vi "NetworkUDP_Recieve.vi"(8 "error in (no error)":errorcluster, 9 "timeout ms (25000)":i32=25000, 10 "IP4 address":u32, 11 "receiver port":u16=5801) -> (0 "error out":errorcluster, 1 "UDP Network Connection out":refnum<k16>, 2 "ConsecErrCount":i32, 3 "data out":string, 4 "SenderAddress":u32)   [LabVIEW 2019, in "Trajectory_Library.lvlib"]
doc: "Listen for and read a packet of data from the network using the UDP protocol. This routine can listen for a single computer or listen for any senders on the subnet. \n\nThis subVI does not return to the caller until either data has been received or a timeout has occured. Suggest putting this function in a separate loop to avoid issues slowing down other code.\n\nInputs:\n -- Receiver Port -- UInt16 -- UDP port number used for listening. Only data sent to this port will be returned. (Optional. Default: 5801)\n -- IP4 Address -- UInt32 -- The IP address of the computer expected to send data. If this value is 0, then then data will be returned for any sender. Use the standard TCP/IP LabVIEW functions to convert a standard IP4 address in the form of 123.123.123.123 to an unsigned integer for this input. (Optional. Default: 0) \n -- Timeout ms -- Int32 -- Timeout value in milliseconds. (Optional. Default: 25000 )\n -- Error in -- Error cluster -- Propagated error cluster. (Optional. Default: no error)\n\nOutputs:\n -- data out -- string -- Last data message sent to the specified port number.\n -- Consec Err -- Int32 -- Counter indicating the number of consecutive errors that have occured.\n -- UDP Network Connection -- UDP Connection Reference -- Reference to the UDP network connection. When finished with communication, the connection should be closed.\n -- Error out -- Error cluster -- Current propagated error cluster."
uses:
  Trajectory_Library.lvlib
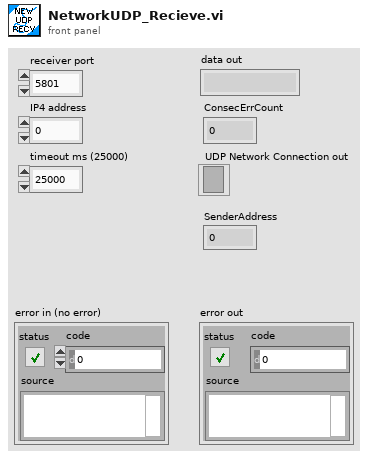
[diagram p1: front panel]
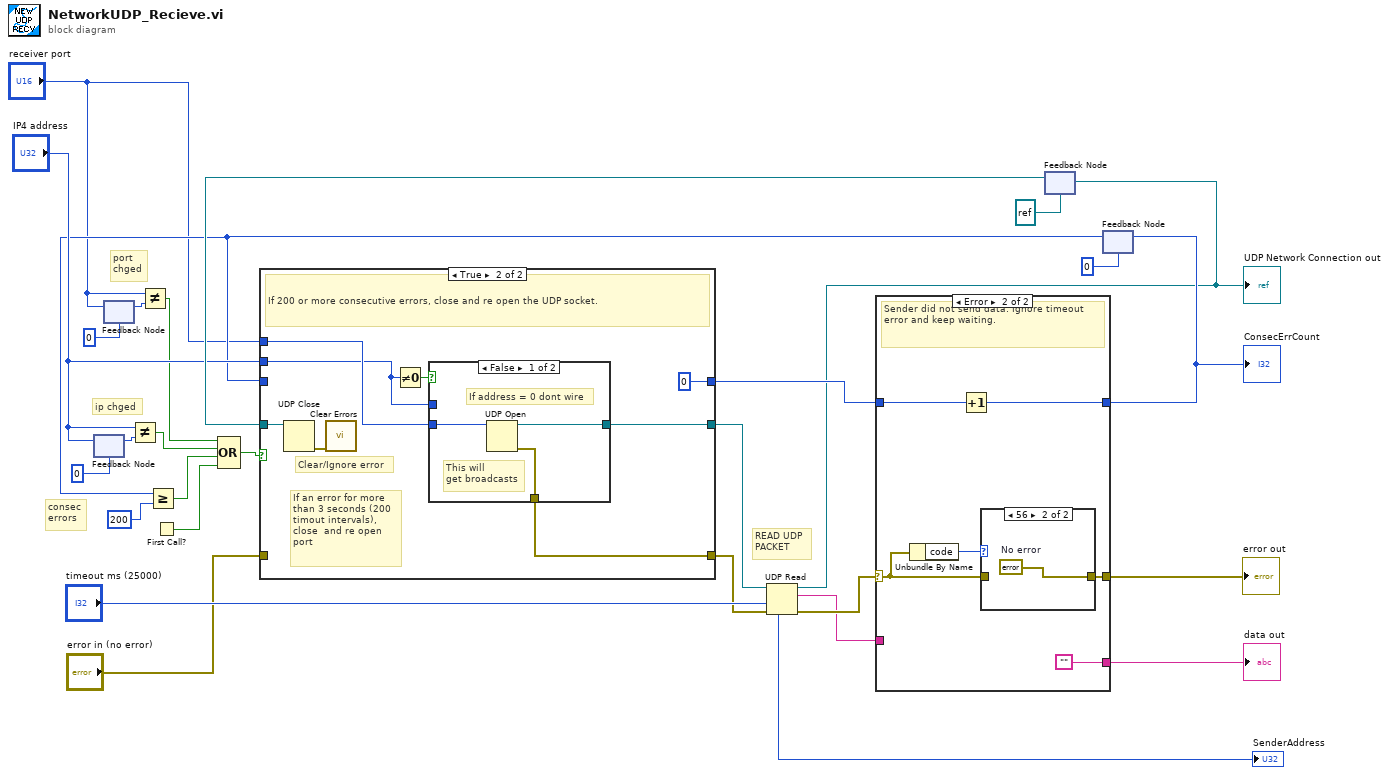
[diagram p0: block diagram]
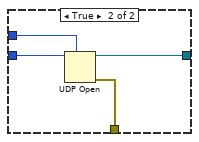
[diagram p3: hidden frame]
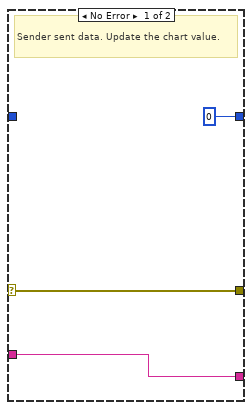
[diagram p4: hidden frame]
diagram:
  # "consec\nerrors"
  # "ip chged"
  # "port\nchged"
  # "READ UDP\nPACKET"
  n1 = feedback-in #1("IP4 address") -> ()
  n2 = feedback #1(u32 0 ("IP4 address")) -> (w15:u32)
  n3 = feedback #2(u16 0 ("receiver port")) -> (w4:u16)
  n4 = feedback-in #2("receiver port") -> ()
  n5 = Not Equal?(x="IP4 address", y=w15) -> (x != y?=w12:bool)
  n6 = Not Equal?(x="receiver port", y=w4) -> (x != y?=w1:bool)
  n7 = First Call?() -> (First Call?: T/F=w9:bool)
  n8 = feedback #3(refnum<k16> refnum ("port")) -> (w22:refnum<k16>)
  n9 = feedback #4(0) -> (w11:i32)
  n10 = Greater Or Equal?(x=w11, y=200) -> (x >= y?=w10:bool)
  n11 = Compound Arithmetic op=OR(w1, w12, w10, w9) -> (w13:bool)
  n12 = case shown="True" w13 {
    tunnel: w11 -> [w31 _]
    tunnel: [w31 0] -> w18
    tunnel: w22 -> [w30 w39]
    tunnel: [w30 w38] -> w21
    tunnel: "error in (no error)" -> [w29 _]
    tunnel: [w29 w37] -> w19
    tunnel: "receiver port" -> [_ w35]
    tunnel: "IP4 address" -> [_ w33]
    frame False {
      # "Not greater than 200 consecutive errors"
    }
    frame True {
      # "Clear/Ignore error"
      # "If an error for more\nthan 3 seconds (200 \ntimout intervals), \nclose  and re open \nport"
      # "If 200 or more consecutive errors, close and re open the UDP socket."
      n13 = UDP Close(connection ID=w39) -> (error out=w32:errorcluster)  [unwired: 1 in, 1 out]
      n14 = call <vilib>:"Clear Errors.vi"("error in (no error)"=w32) -> ()  [unwired: 5 in, 2 out]
      n15 = Not Equal To 0?(x=w33) -> (x != 0?=w34:bool)
      n16 = case shown="False" w34 {
        tunnel: [w41 w46] -> w38
        tunnel: [w42 w45] -> w37
        tunnel: w35 -> [w40 w44]
        tunnel: w33 -> [_ w43]
        frame False {
          # "This will\nget broadcasts"
          # "If address = 0 dont wire"
          n17 = UDP Open(11:w40) -> (port=w41:refnum<k16>, 0:w42:errorcluster)  [unwired: 4 in, 1 out]
        }
        frame True {
          n18 = UDP Open(7:w43, 11:w44) -> (port=w46:refnum<k16>, 0:w45:errorcluster)  [unwired: 3 in, 1 out]
        }
      }
    }
  }
  n19 = UDP Read(connection ID=w21, timeout ms (25000)="timeout ms (25000)", 8:w19) -> (data out=w26:string, error out=w27:errorcluster, 3:w6:refnum<k16>, 6:→"SenderAddress":u32)  [unwired: 2 out]
  "UDP Network Connection out" <- w6
  n20 = case shown="Error" w27 {
    selector: w27 -> [w49 w54]
    tunnel: w26 -> [w48 _]
    tunnel: [w49 w53] -> w5
    tunnel: w18 -> [_ w52]
    tunnel: [w48 ""] -> w8
    tunnel: [0 w51] -> w7
    frame No Error {
      (unwired) 0
      # "Sender sent data. Update the chart value."
    }
    frame Error {
      # "Sender did not send data. Ignore timeout error and keep waiting."
      n21 = Unbundle By Name(w54) -> ("code"=w55:i32)
      n22 = Increment(x=w52) -> (x+1=w51:i32)
      n23 = case shown="56" w55 {
        tunnel: w54 -> [w56 _]
        tunnel: [w56 w57] -> w53
        frame Default {
        }
        frame 56 {
          w57 = errorcluster {"status"=FALSE, "code"=0, "source"=""}  # No error
        }
      }
    }
  }
  "error out" <- w5
  "ConsecErrCount" <- w7
  "data out" <- w8
  n24 = feedback-in #3(w6) -> ()
  n25 = feedback-in #4(w7) -> ()
